vi "ReplacePolySubVINode.vi"(5 "Old File Name":string="PolyA String.vi", 7 "New File Name":string="PolyB.vi", 8 "error in (no error)":errorcluster, 11 "VI Refnum":refnum<vi>) -> (0 "error out":errorcluster, 3 "VI Refnum Out":refnum<vi>, 4 "Replaced":bool)   [LabVIEW 2024]
uses:
  <vilib>/Utility/traverseref.llb/TRef TravTarget.ctl
  <vilib>/Utility/traverseref.llb/VI Scripting - Traverse.lvlib
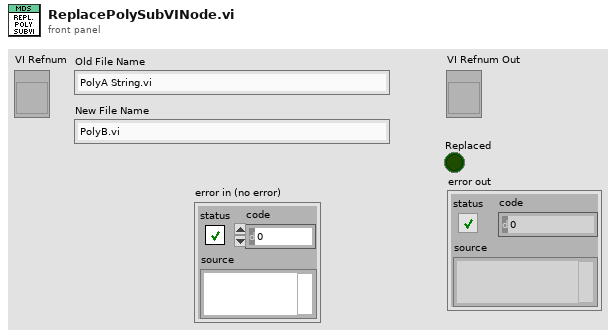
[diagram p1: front panel]
types:
  T1 = typedef "TRef TravTarget.ctl" = enum16{"FP", "BD", "Other"}
  T2 = cluster{"VIPath":path, "Menu Name":string, "Selector Name":string}[]
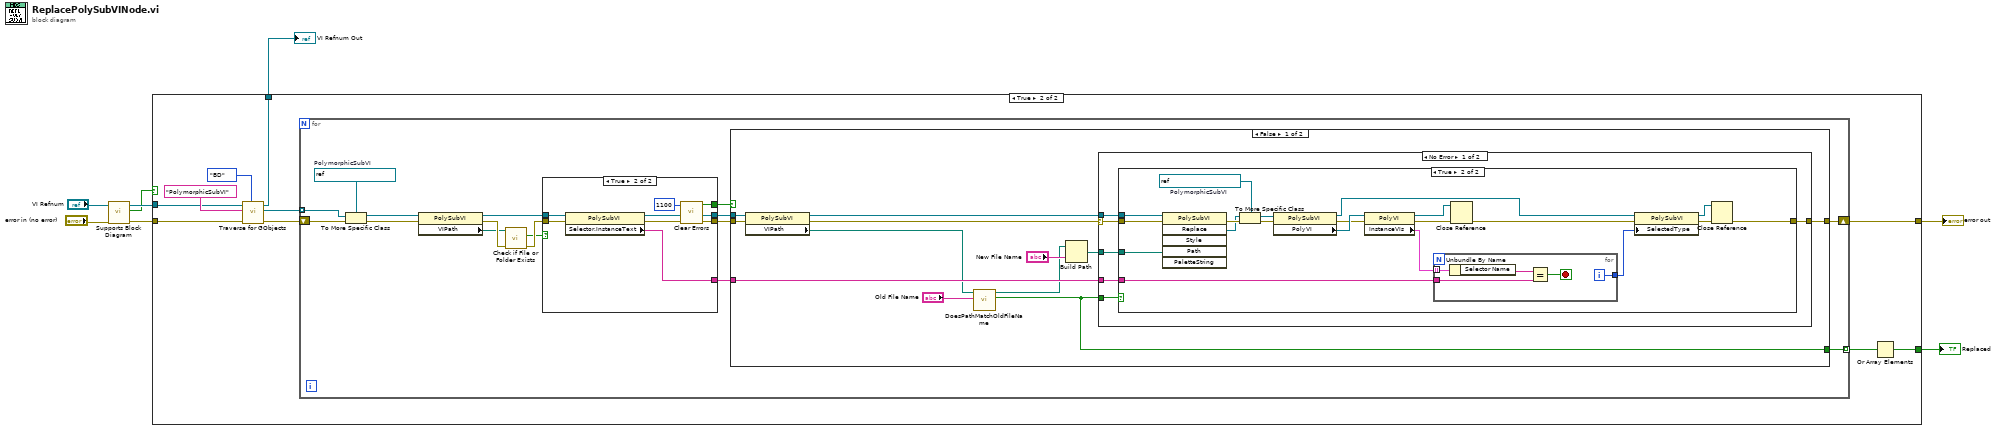
[diagram p0: block diagram]
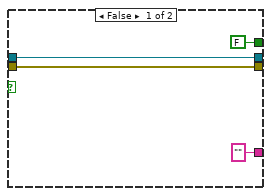
[diagram p3: hidden frame]
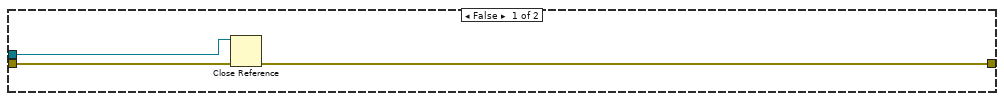
[diagram p4: hidden frame]
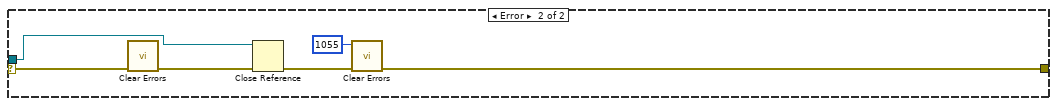
[diagram p5: hidden frame]
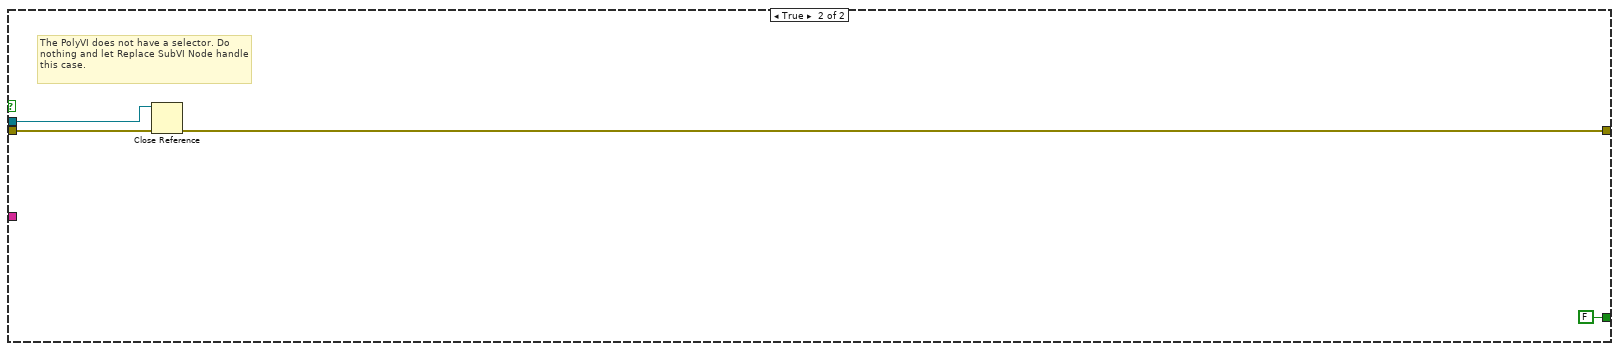
[diagram p6: hidden frame]
diagram:
  n1 = call "Supports Block Diagram.vi"("error in (no error)"="error in (no error)", "vi in"="VI Refnum") -> ("error out"=w6:errorcluster, "has block diagram"=w5:bool, "vi out"=w7:refnum<vi>)  [unwired: 7 in]
  n2 = case shown="True" w5 {
    tunnel: [_ w11] -> w8
    tunnel: [w9 w16] -> w1
    tunnel: w7 -> [w10 w15]
    tunnel: w6 -> [w9 w14]
    tunnel: [w10 w13] -> w2
    frame False {
    }
    frame True {
      n3 = call <vilib>:"Traverse for GObjects.vi"("Traverse Target"=TRef_TravTarget."BD", "error in (no error)"=w14, "Class Name"="PolymorphicSubVI", "VI Refnum"=w15) -> ("error out"=w19:errorcluster, "References"=w20:refnum<vi>[], "dup VI Refnum"=w13:refnum<vi>)  [unwired: 4 in, 1 out]
      n4 = for {
        shift-right: [w33] -> w16
        shift-left: w19 -> [w34]
        tunnel: w20 -> [w35] mode=indexing
        tunnel: [w30] -> w12 mode=indexing
        w36 = refnum<vi> refnum  # PolymorphicSubVI
        n5 = To More Specific Class(target class=w36, reference=w35, error in=w34) -> (specific class reference=w27:refnum<vi>, error out=w25:errorcluster)
        n6 = property class="PolySubVI"(reference=w27, error in=w25) -> (reference out=w26:refnum<vi>, error out=w24:errorcluster, "VIPath"=w22:path)
        n7 = call <vilib>:"Check if File or Folder Exists.vi"("error in (no error)"=w24, "path"=w22) -> ("error out"=w23:errorcluster, "file or folder exists?"=w21:bool)  [unwired: 7 in, 1 out]
        n8 = case shown="True" w21 {
          tunnel: [w40 w48] -> w32
          tunnel: ["" ("Selector.InstanceText") w47] -> w31
          tunnel: [w37 w45] -> w29
          tunnel: [FALSE ("specific error cleared?") w43] -> w28
          tunnel: w26 -> [w40 w42]
          tunnel: w23 -> [w37 w41]
          frame False {
          }
          frame True {
            n9 = property class="PolySubVI"(reference=w42, error in=w41) -> (reference out=w48:refnum<vi>, error out=w46:errorcluster, "Selector.InstanceText"=w47:string)
            n10 = call <vilib>:"Clear Errors.vi"("error in (no error)"=w46, "specific error code to clear (0: all)"=1100) -> ("error out"=w45:errorcluster, "specific error cleared?"=w43:bool)  [unwired: 4 in]
          }
        }
        n11 = case shown="False" w28 {
          tunnel: [w60 w103] -> w33
          tunnel: w32 -> [w57 w102]
          tunnel: w31 -> [w56 _]
          tunnel: [w54 FALSE ("Match Found")] -> w30
          tunnel: w29 -> [w52 w104]
          frame False {
            n12 = property class="PolySubVI"(reference=w57, error in=w52) -> (reference out=w49:refnum<vi>, error out=w50:errorcluster, "VIPath"=w51:path)
            n13 = call "DoesPathMatchOldFileName.vi"("Old File Name"="Old File Name", "File Path"=w51) -> ("Match Found"=w54:bool, "Parent Directory"=w53:path)  [unwired: 8 in]
            n14 = Build Path(base path=w53, name or relative path="New File Name") -> (appended path=w58:path)
            n15 = case shown="No Error" w50 {
              selector: w50 -> [w62 w100]
              tunnel: w58 -> [w66 _]
              tunnel: w54 -> [w65 _]
              tunnel: [w64 w96] -> w60
              tunnel: w49 -> [w63 w98]
              tunnel: w56 -> [w61 _]
              frame No Error {
                n16 = case shown="True" w65 {
                  tunnel: w66 -> [_ w70]
                  tunnel: w62 -> [w69 w89]
                  tunnel: [w68 w72] -> w64
                  tunnel: w63 -> [w67 w88]
                  tunnel: w61 -> [_ w81]
                  frame False {
                    n17 = Close Reference(reference=w67, error in (no error)=w69) -> (error out=w68:errorcluster)
                  }
                  frame True {
                    w87 = refnum<vi> refnum  # PolymorphicSubVI
                    n18 = invoke class="PolySubVI" method="Replace"(reference=w88, error in=w89, "Path"=w70) -> (error out=w86:errorcluster, "Replace"=w71:refnum<vi>)  [unwired: 3 in, 4 out]
                    n19 = To More Specific Class(target class=w87, reference=w71, error in=w86) -> (specific class reference=w84:refnum<vi>, error out=w85:errorcluster)
                    n20 = property class="PolySubVI"(reference=w84, error in=w85) -> (reference out=w79:refnum<vi>, error out=w80:errorcluster, "PolyVI"=w83:refnum<vi>)
                    n21 = property class="PolyVI"(reference=w83, error in=w80) -> (reference out=w75:refnum<vi>, error out=w77:errorcluster, "InstanceVIs"=w82:T2)
                    n22 = for {
                      tunnel: w82 -> [w93] mode=indexing
                      tunnel: w81 -> [w94]
                      tunnel: [w90] -> w78
                      i -> [w90]
                      stop <- w91 stop-if-true
                      n23 = Unbundle By Name(w93) -> ("Selector Name"=w92:string)
                      n24 = Equal?(x=w92, y=w94) -> (x = y?=w91:bool)
                    }
                    n25 = Close Reference(reference=w75, error in (no error)=w77) -> (error out=w76:errorcluster)
                    n26 = property class="PolySubVI"(reference=w79, error in=w76, "SelectedType"=w78) -> (reference out=w73:refnum<vi>, error out=w74:errorcluster)
                    n27 = Close Reference(reference=w73, error in (no error)=w74) -> (error out=w72:errorcluster)
                  }
                }
              }
              frame Error {
                n28 = call <vilib>:"Clear Errors.vi"("error in (no error)"=w100) -> ("error out"=w99:errorcluster)  [unwired: 5 in, 1 out]
                n29 = Close Reference(reference=w98, error in (no error)=w99) -> (error out=w97:errorcluster)
                n30 = call <vilib>:"Clear Errors.vi"("error in (no error)"=w97, "specific error code to clear (0: all)"=1055) -> ("error out"=w96:errorcluster)  [unwired: 4 in, 1 out]
              }
            }
          }
          frame True {
            # "The PolyVI does not have a selector. Do nothing and let Replace SubVI Node handle this case."
            n31 = Close Reference(reference=w102, error in (no error)=w104) -> (error out=w103:errorcluster)
          }
        }
      }
      n32 = Or Array Elements(Boolean array=w12) -> (logical OR=w11:bool)
    }
  }
  "error out" <- w1
  "Replaced" <- w8
  "VI Refnum Out" <- w2
